vi "RT Timestamp Delta Analysis.vi"(4 "warmup iterations":i32=10, 6 "calibration array":u64[](array[numeric]), 8 "error in (no error)":errorcluster, 10 "timestamp array 2":u64[](array[numeric]), 11 "timestamp array 1":u64[](array[numeric])) -> (0 "error out":errorcluster, 1 "max jitter (uS)":dbl format="%.2f", 2 "execution histogram":T1(graph), 3 "execution times (uS)":dbl[](graph), 5 "standard deviation (uS)":dbl format="%.2f", 7 "mean time (uS)":dbl format="%.2f")   [LabVIEW 2013]
doc: "Analyzes the array of timestamps returned by the RT Get Timestamp VI."
uses:
  <vilib>/Analysis/NI_AALBase.lvlib
  <vilib>/Analysis/baseanly.llb/Mean (DBL).vi
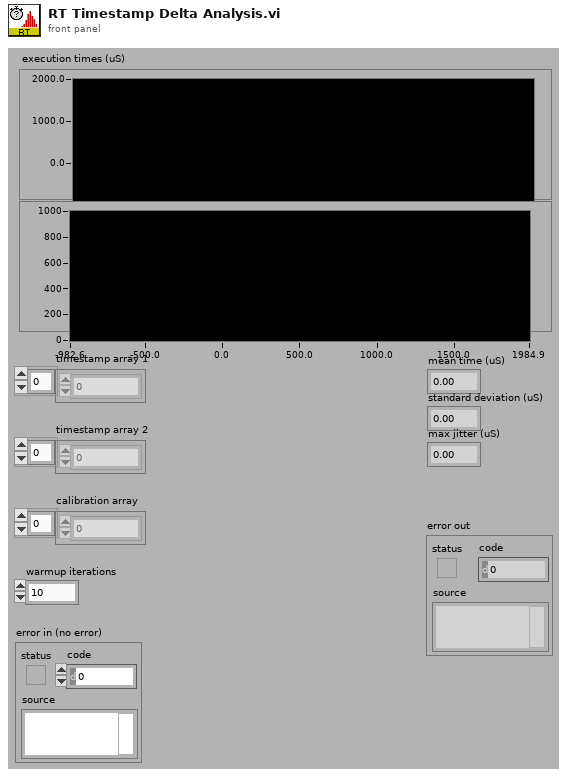
[diagram p1: front panel]
types:
  T1 = cluster{"X Values":dbl[], "Histogram: h(x)":i32[]}
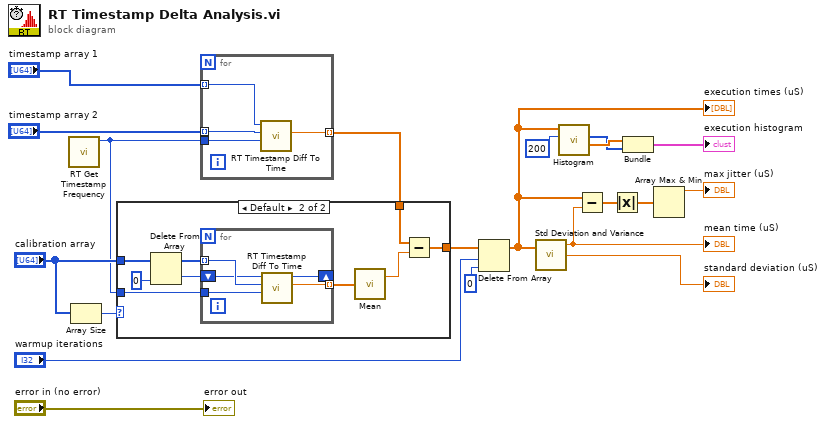
[diagram p0: block diagram]
diagram:
  n1 = call <vilib>:"RT Get Timestamp Frequency.vi"() -> ("timestamp frequency (Hz)"=w10:u32)  [unwired: 1 in, 10 out]
  n2 = Array Size(array="calibration array") -> (size(s)=w11:i32)
  n3 = for {
    tunnel: [w23] -> w14 mode=indexing
    tunnel: w10 -> [w24]
    tunnel: "timestamp array 1" -> [w22] mode=indexing
    tunnel: "timestamp array 2" -> [w21] mode=indexing
    n4 = call <vilib>:"RT Timestamp Diff To Time.vi"("timestamp frequency (Hz)"=w24, "t2"=w21, "t1"=w22) -> ("t2-t1 (uS)"=w23:dbl)  [unwired: 4 in, 4 out]
  }
  n5 = case shown="Default" w11 {
    tunnel: "calibration array" -> [_ w31]
    tunnel: [w25 w33] -> w13
    tunnel: w14 -> [w25 w34]
    tunnel: w10 -> [_ w26]
    frame 0 {
    }
    frame Default {
      n6 = Delete From Array(array=w31, index=0) -> (deleted portion=w30:u64, array with subset deleted=w29:u64[])  [unwired: 1 in]
      n7 = for {
        shift-right: [w38] -> _
        shift-left: w30 -> [w35]
        tunnel: w29 -> [w36] mode=indexing
        tunnel: [w39] -> w27 mode=indexing
        tunnel: w26 -> [w37]
        n8 = call <vilib>:"RT Timestamp Diff To Time.vi"("timestamp frequency (Hz)"=w37, "t2"=w36, "t1"=w35) -> ("t2-t1 (uS)"=w39:dbl, "dup t2"=w38:u64)  [unwired: 3 in, 4 out]
      }
      n9 = call-poly <vilib>:"Mean.vi"("X"=w27) -> ("mean"=w28:dbl)  [unwired: 1 out]
      n10 = Subtract(x=w34, y=w28) -> (x-y=w33:dbl[])
    }
  }
  n11 = Delete From Array(array=w13, length="warmup iterations", index=0) -> (array with subset deleted=w5:dbl[])  [unwired: 1 out]
  "execution times (uS)" <- w5
  n12 = call <vilib>:"Std Deviation and Variance.vi"("X"=w5) -> ("mean"=w4:dbl, "standard deviation"=→"standard deviation (uS)":dbl)  [unwired: 1 in, 1 out]
  "mean time (uS)" <- w4
  n13 = call <vilib>:"Histogram.vi"("intervals"=200, "X"=w5) -> ("X Values"=w17:dbl[], "Histogram: h(x)"=w16:i32[])  [unwired: 8 out]
  n14 = Subtract(x=w5, y=w4) -> (x-y=w19:dbl[])
  n15 = Absolute Value(x=w19) -> (abs(x)=w18:dbl[])
  n16 = Bundle("X Values"=w17, "Histogram: h(x)"=w16) -> (→"execution histogram":T1)  [unwired: 1 out]
  n17 = Array Max & Min(array=w18) -> (max value=→"max jitter (uS)":dbl)  [unwired: 3 out]
  "error out" <- "error in (no error)"
